vi "Waveform Data Convert.vi"(5 "Input Data":string, 9 "Range":dbl format="%.2f") -> (6 "Output":dbl[](array[numeric]) format="%.2f", 8 "Precision":i16, 10 "Data Byte Number":i32)   [LabVIEW 2014, in "Yokogawa.lvlib" / "Yokogawa PZ4000.lvlib"]
doc: "This VI transforms acquisition word string data into voltage array values for the Waveform Graph."
uses:
  Yokogawa PZ4000.lvlib
panel:
  # "(INPUT - 2048)\n OUTPUT = ( -------------- x RANGE ) \n                         2048"
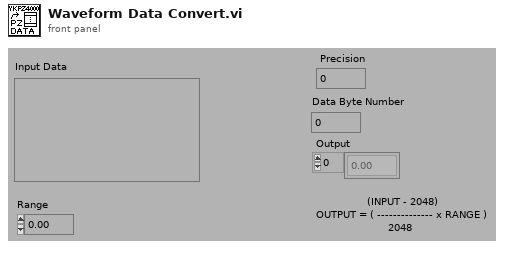
[diagram p1: front panel]
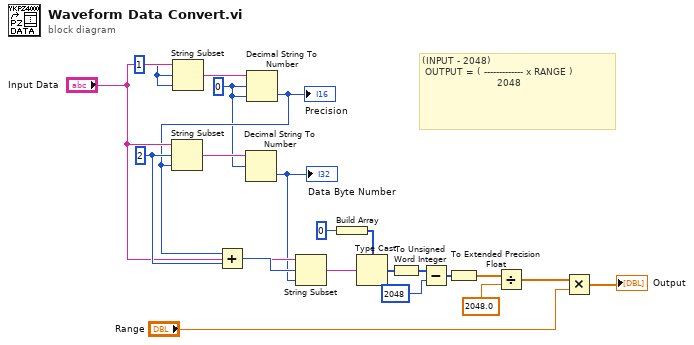
[diagram p0: block diagram]
diagram:
  w21 = 2
  w14 = 1
  w5 = i16 0
  # "(INPUT - 2048)\n OUTPUT = ( ------------- x RANGE ) \n                         2048"
  n1 = String Subset(string="Input Data", offset (0)=w14, length (rest)=w14) -> (substring=w19:string)
  n2 = Decimal String To Number(string=w19, offset=w5, default (0L)=w5) -> (number=w16:i16)  [unwired: 1 out]
  "Precision" <- w16
  n3 = String Subset(string="Input Data", offset (0)=w21, length (rest)=w16) -> (substring=w20:string)
  n4 = Add(x=w16, y=w21) -> (x+y=w18:i32)
  n5 = Decimal String To Number(string=w20, offset=w5) -> (number=w15:i32)  [unwired: 1 in, 1 out]
  "Data Byte Number" <- w15
  n6 = String Subset(string="Input Data", offset (0)=w18, length (rest)=w15) -> (substring=w7:string)
  n7 = Build Array(i16 0) -> (w12:i16[])
  n8 = Type Cast(type=w12, x=w7) -> (*(type *) &x=w10:i16[])
  n9 = To Unsigned Word Integer(number=w10) -> (unsigned 16bit integer=w8:u16[])
  n10 = Subtract(x=w8, y=2048) -> (x-y=w9:i32[])
  n11 = To Extended Precision Float(1:w9) -> (0:w3:ext[])
  n12 = Divide(x=w3, y=2048.0) -> (x/y=w4:ext[])
  n13 = Multiply(x=w4, y="Range") -> (x*y=→"Output":ext[])
